vi "CreateSwapArray_v2.vi"(8 "error in (no error)":errorcluster, 9 "ROSCO Params":T3, 10 "Index In":T2={"iSTATUS"=0, "TIME"=0, "DT"=0, "BL_PITCH_1"=0, "VS_MECHGENPWR"=13, "GEN_SPEED"=0, "ROT_SPEED"=0, "GENTQMEAS"=0, "Y_M"=0, "HORWINDV"=0, "ROOTMOOP1"=0, "ROOTMOOP2"=0, "BL_PITCH_2"=0, "BL_PITCH_3"=0, "ROOTMOOP3"=0, "INFILE_SIZE"=0, "FA_ACC"=0, "NUM_BLADES"=0, " OUT BL_PITCH"=0, "OUT_ TORQUE"=0, "OUTFILE_SIZE "=0, "AVCMSG_SIZE"=0, "AERODYN TQ"=46, "VS_GENPWR"=0}, 11 "SwapIn":T1) -> (0 "error out":errorcluster, 1 "ROSCO Params Out":T3, 2 "Index Out":T2={"iSTATUS"=0, "TIME"=0, "DT"=0, "BL_PITCH_1"=0, "VS_MECHGENPWR"=13, "GEN_SPEED"=0, "ROT_SPEED"=0, "GENTQMEAS"=0, "Y_M"=0, "HORWINDV"=0, "ROOTMOOP1"=0, "ROOTMOOP2"=0, "BL_PITCH_2"=0, "BL_PITCH_3"=0, "ROOTMOOP3"=0, "INFILE_SIZE"=0, "FA_ACC"=0, "NUM_BLADES"=0, " OUT BL_PITCH"=0, "OUT_ TORQUE"=0, "OUTFILE_SIZE "=0, "AVCMSG_SIZE"=0, "AERODYN TQ"=46, "VS_GENPWR"=0}, 3 "SwapIn Out":T1, 4 "avrSWAP":sgl[](array[numeric]))   [LabVIEW 2018]
uses:
  Clusters/SwapIn.ctl
  Clusters/SwapIndexes.ctl
  Clusters/RoscoParams.ctl
  Clusters/ArrayPairs.ctl
  Clusters/SwapArrayCluster.ctl
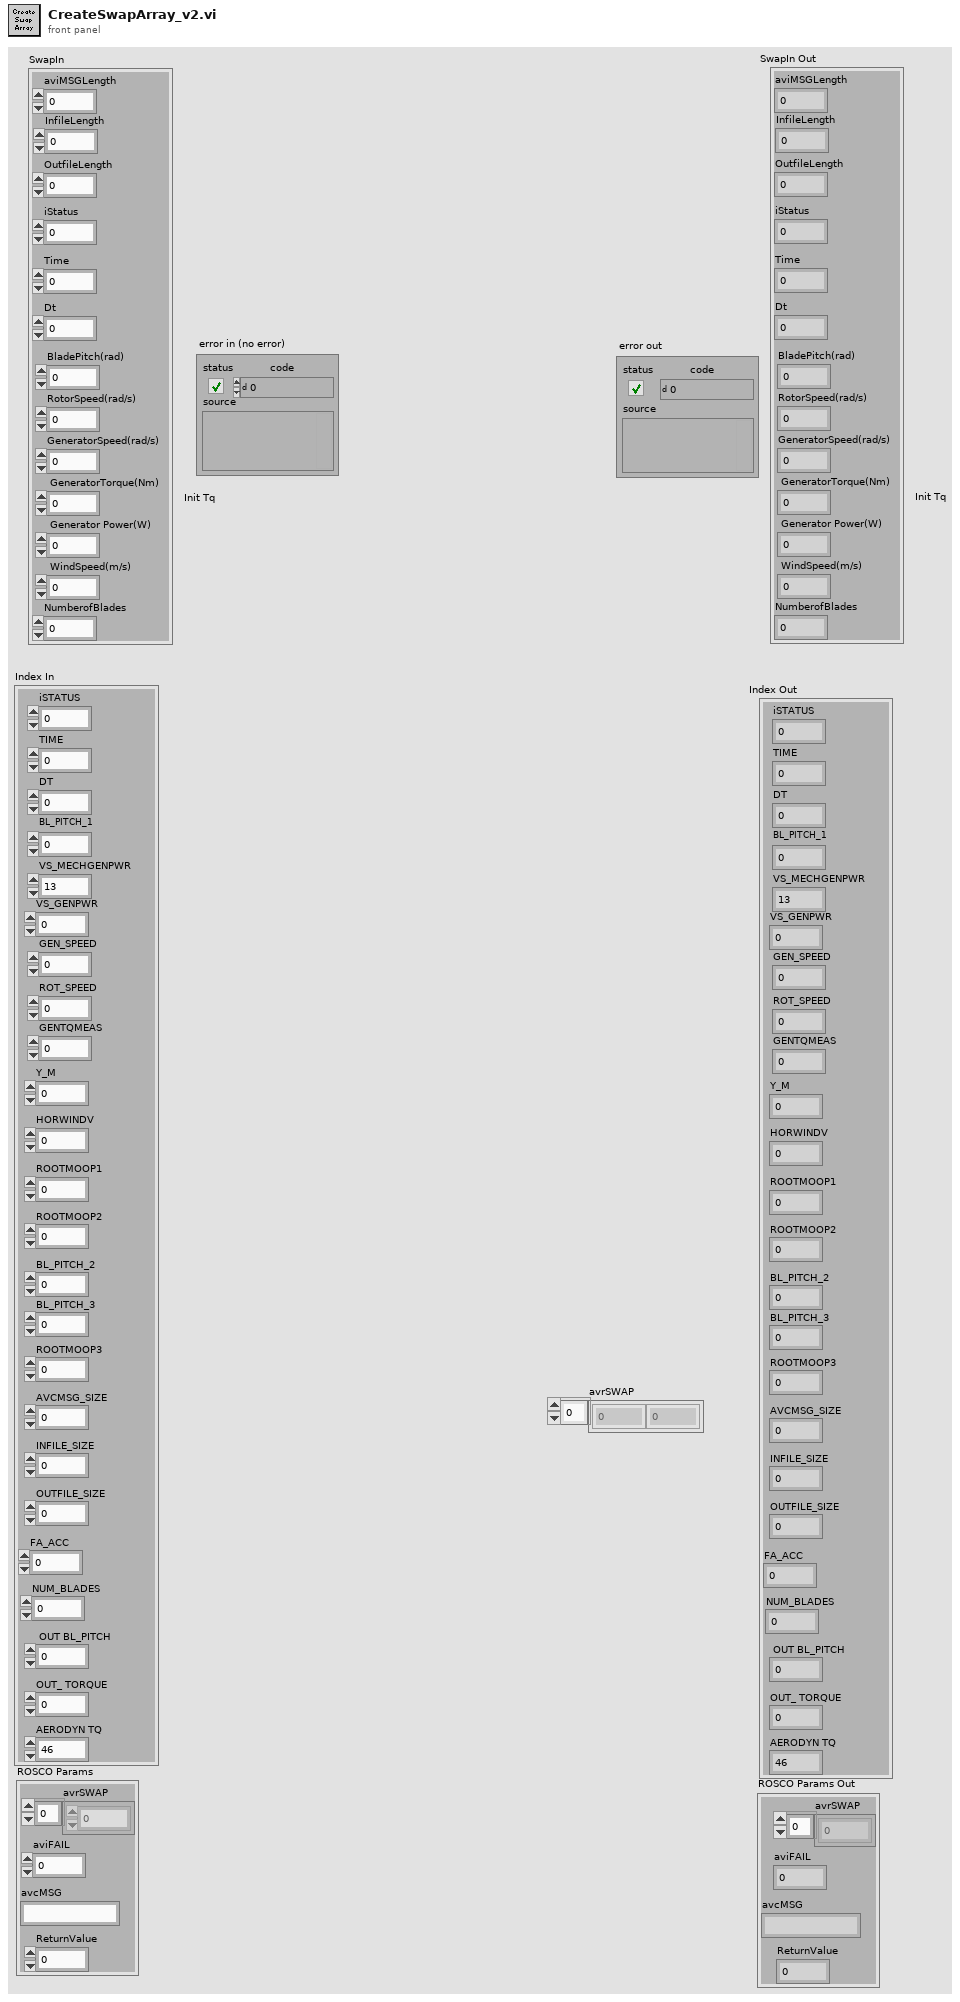
[diagram p1: front panel]
types:
  T1 = typedef "SwapIn.ctl" = cluster{"BladePitch(rad)":sgl, "RotorSpeed(rad/s)":sgl, "GeneratorSpeed(rad/s)":sgl, " GeneratorTorque(Nm)":sgl, " Generator Power(W) ":sgl, " WindSpeed(m/s)":sgl, "aviMSGLength":sgl, "InfileLength":sgl, "OutfileLength":sgl, "iStatus":sgl, "Time":sgl, "Dt":sgl, "NumberofBlades":sgl}
  T2 = typedef "SwapIndexes.ctl" = cluster{"iSTATUS":i32, "TIME":i32, "DT":i32, "BL_PITCH_1":i32, "VS_MECHGENPWR":i32, "GEN_SPEED":i32, "ROT_SPEED":i32, "GENTQMEAS":i32, "Y_M":i32, "HORWINDV":i32, "ROOTMOOP1":i32, "ROOTMOOP2":i32, "BL_PITCH_2":i32, "BL_PITCH_3":i32, "ROOTMOOP3":i32, "INFILE_SIZE":i32, "FA_ACC":i32, "NUM_BLADES":i32, " OUT BL_PITCH":i32, "OUT_ TORQUE":i32, "OUTFILE_SIZE ":i32, "AVCMSG_SIZE":i32, "AERODYN TQ":i32, "VS_GENPWR":i32}
  T3 = typedef "RoscoParams.ctl" = cluster{"avrSWAP":sgl[], "aviFAIL":i32, "avcMSG":string, "ReturnValue":i32}
  T4 = typedef "ArrayPairs.ctl" = cluster{"iStatus":T5, "TIME":T5, "DT":T5, "BL_PITCH":T5, "VS_MECHGENPWR":T5, "VS_GENPWR":T5, "GEN_SPEED":T5, "ROTOR_SPEED":T5, "GENTQMEAS":T5, "Y_M":T5, "HORWINDV":T5, "ROOTMOOP1":T5, "ROOTMOOP2":T5, "BL_PITCH2":T5, "BL_PITCH3":T5, "ROOTMOOP3":T5, "AVCMSG_SIZE":T5, "INFILE_SIZE ":T5, "OUTFILE_SIZE ":T5, "FA_ACC":T5, "NUM_BLADES":T5, "OUT_BL_PITCH":T5, "OUT_TORQUE":T5, "OUT_AERODYN_TQ":T5}
  T5 = typedef "SwapArrayCluster.ctl" = cluster{"Index":i32, "Value":sgl}
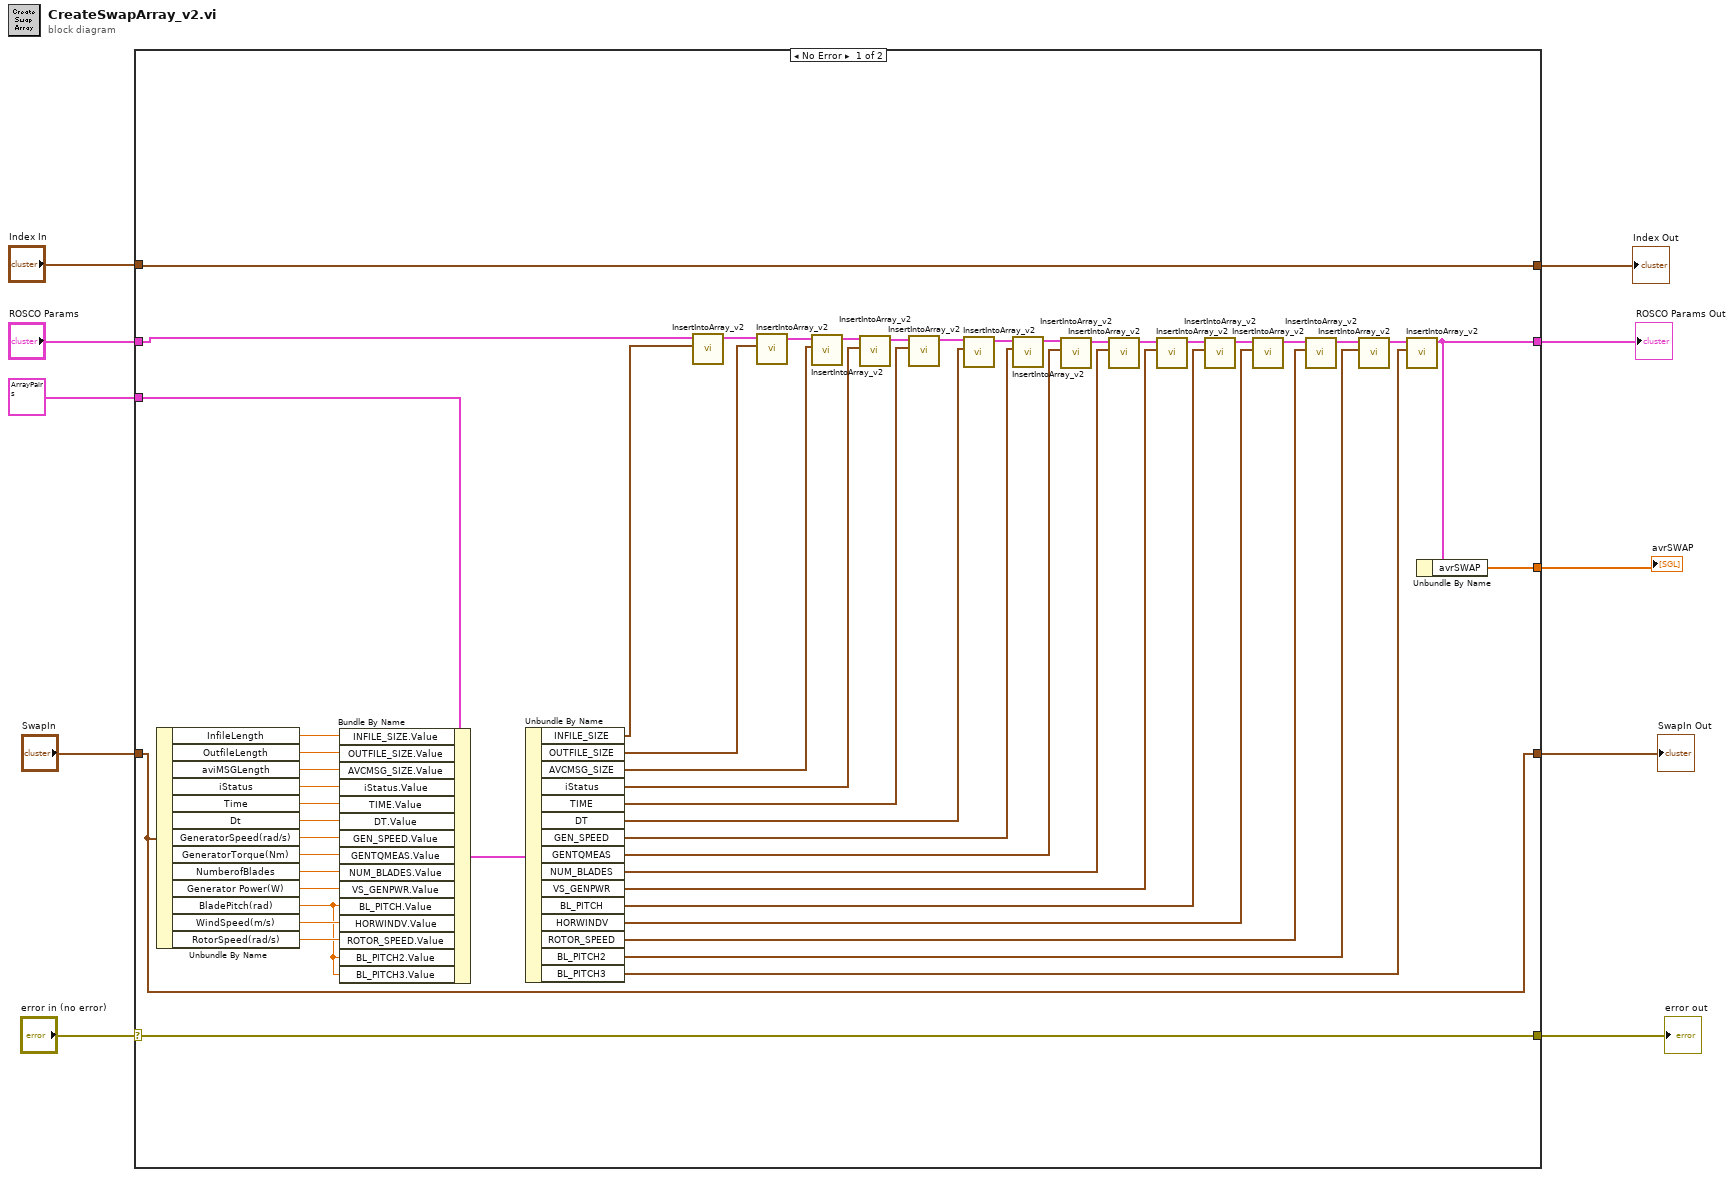
[diagram p0: block diagram]
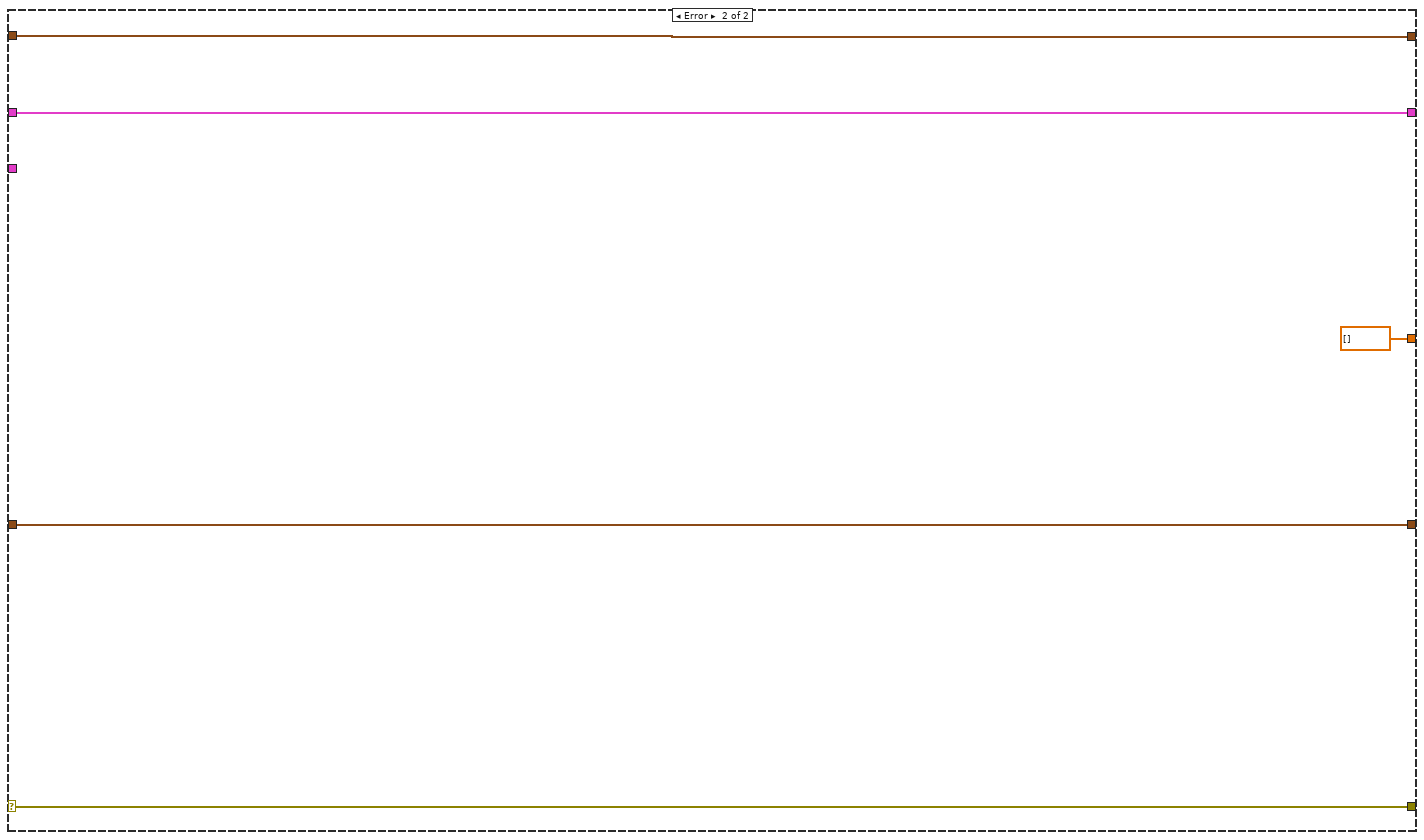
[diagram p2: hidden frame]
diagram:
  n1 = case shown="No Error" "error in (no error)" {
    selector: "error in (no error)" -> [w17 w62]
    tunnel: "SwapIn" -> [w59 w63]
    tunnel: "Index In" -> [w60 w64]
    tunnel: "ROSCO Params" -> [w46 w65]
    tunnel: [w60 w64] -> w7
    tunnel: [w11 w65] -> w6
    tunnel: [w59 w63] -> w5
    tunnel: T4 {"iStatus"={"Index"=0, "Value"=0.0}, "TIME"={"Index"=1, "Value"=0.0}, "DT"={"Index"=2, "Value"=0.0}, "BL_PITCH"={"Index"=3, "Value"=0.0}, "VS_MECHGENPWR"={"Index"=13, "Value"=0.0}, "VS_GENPWR"={"Index"=14, "Value"=0.0}, "GEN_SPEED"={"Index"=19, "Value"=0.0}, "ROTOR_SPEED"={"Index"=20, "Value"=0.0}, "GENTQMEAS"={"Index"=22, "Value"=0.0}, "Y_M"={"Index"=23, "Value"=0.0}, "HORWINDV"={"Index"=26, "Value"=0.0}, "ROOTMOOP1"={"Index"=29, "Value"=0.0}, "ROOTMOOP2"={"Index"=30, "Value"=0.0}, "BL_PITCH2"={"Index"=32, "Value"=0.0}, "BL_PITCH3"={"Index"=33, "Value"=0.0}, "ROOTMOOP3"={"Index"=31, "Value"=0.0}, "AVCMSG_SIZE"={"Index"=48, "Value"=0.0}, "INFILE_SIZE "={"Index"=49, "Value"=0.0}, "OUTFILE_SIZE "={"Index"=50, "Value"=0.0}, "FA_ACC"={"Index"=52, "Value"=0.0}, "NUM_BLADES"={"Index"=60, "Value"=0.0}, "OUT_BL_PITCH"={"Index"=44, "Value"=0.0}, "OUT_TORQUE"={"Index"=46, "Value"=0.0}, "OUT_AERODYN_TQ"={"Index"=89, "Value"=0.0}} ("ArrayPairs") -> [w45 _]
    tunnel: [w17 w62] -> w3
    tunnel: [w18 sgl[] [] ("avrSWAP")] -> w1
    frame No Error {
      n2 = Unbundle By Name(w59) -> ("InfileLength"=w47:sgl, "OutfileLength"=w48:sgl, "aviMSGLength"=w49:sgl, "iStatus"=w50:sgl, "Time"=w51:sgl, "Dt"=w52:sgl, "GeneratorSpeed(rad/s)"=w53:sgl, "GeneratorTorque(Nm)"=w54:sgl, "NumberofBlades"=w55:sgl, "Generator Power(W)"=w56:sgl, "BladePitch(rad)"=w16:sgl, "WindSpeed(m/s)"=w57:sgl, "RotorSpeed(rad/s)"=w58:sgl)
      n3 = Bundle By Name(cluster=w45, "INFILE_SIZE.Value"=w47, "OUTFILE_SIZE.Value"=w48, "AVCMSG_SIZE.Value"=w49, "iStatus.Value"=w50, "TIME.Value"=w51, "DT.Value"=w52, "GEN_SPEED.Value"=w53, "GENTQMEAS.Value"=w54, "NUM_BLADES.Value"=w55, "VS_GENPWR.Value"=w56, "BL_PITCH.Value"=w16, "HORWINDV.Value"=w57, "ROTOR_SPEED.Value"=w58, "BL_PITCH2.Value"=w16, "BL_PITCH3.Value"=w16) -> (w44:T4)
      n4 = Unbundle By Name(w44) -> ("INFILE_SIZE"=w43:T5, "OUTFILE_SIZE"=w37:T5, "AVCMSG_SIZE"=w35:T5, "iStatus"=w34:T5, "TIME"=w33:T5, "DT"=w26:T5, "GEN_SPEED"=w25:T5, "GENTQMEAS"=w24:T5, "NUM_BLADES"=w23:T5, "VS_GENPWR"=w22:T5, "BL_PITCH"=w21:T5, "HORWINDV"=w20:T5, "ROTOR_SPEED"=w19:T5, "BL_PITCH2"=w15:T5, "BL_PITCH3"=w14:T5)
      n5 = call "InsertIntoArray_v2.vi"("ROSCO Params"=w46, "KeyVal"=w43) -> ("ROSCO Params Out"=w42:T3)  [unwired: 7 in, 1 out]
      n6 = call "InsertIntoArray_v2.vi"("ROSCO Params"=w42, "KeyVal"=w37) -> ("ROSCO Params Out"=w36:T3)  [unwired: 7 in, 1 out]
      n7 = call "InsertIntoArray_v2.vi"("ROSCO Params"=w36, "KeyVal"=w35) -> ("ROSCO Params Out"=w32:T3)  [unwired: 7 in, 1 out]
      n8 = call "InsertIntoArray_v2.vi"("ROSCO Params"=w32, "KeyVal"=w34) -> ("ROSCO Params Out"=w41:T3)  [unwired: 7 in, 1 out]
      n9 = call "InsertIntoArray_v2.vi"("ROSCO Params"=w41, "KeyVal"=w33) -> ("ROSCO Params Out"=w31:T3)  [unwired: 7 in, 1 out]
      n10 = call "InsertIntoArray_v2.vi"("ROSCO Params"=w31, "KeyVal"=w26) -> ("ROSCO Params Out"=w40:T3)  [unwired: 7 in, 1 out]
      n11 = call "InsertIntoArray_v2.vi"("ROSCO Params"=w40, "KeyVal"=w25) -> ("ROSCO Params Out"=w30:T3)  [unwired: 7 in, 1 out]
      n12 = call "InsertIntoArray_v2.vi"("ROSCO Params"=w30, "KeyVal"=w24) -> ("ROSCO Params Out"=w39:T3)  [unwired: 7 in, 1 out]
      n13 = call "InsertIntoArray_v2.vi"("ROSCO Params"=w39, "KeyVal"=w23) -> ("ROSCO Params Out"=w29:T3)  [unwired: 7 in, 1 out]
      n14 = call "InsertIntoArray_v2.vi"("ROSCO Params"=w29, "KeyVal"=w22) -> ("ROSCO Params Out"=w28:T3)  [unwired: 7 in, 1 out]
      n15 = call "InsertIntoArray_v2.vi"("ROSCO Params"=w28, "KeyVal"=w21) -> ("ROSCO Params Out"=w38:T3)  [unwired: 7 in, 1 out]
      n16 = call "InsertIntoArray_v2.vi"("ROSCO Params"=w38, "KeyVal"=w20) -> ("ROSCO Params Out"=w27:T3)  [unwired: 7 in, 1 out]
      n17 = call "InsertIntoArray_v2.vi"("ROSCO Params"=w27, "KeyVal"=w19) -> ("ROSCO Params Out"=w13:T3)  [unwired: 7 in, 1 out]
      n18 = call "InsertIntoArray_v2.vi"("ROSCO Params"=w13, "KeyVal"=w15) -> ("ROSCO Params Out"=w12:T3)  [unwired: 7 in, 1 out]
      n19 = call "InsertIntoArray_v2.vi"("ROSCO Params"=w12, "KeyVal"=w14) -> ("ROSCO Params Out"=w11:T3)  [unwired: 7 in, 1 out]
      n20 = Unbundle By Name(w11) -> ("avrSWAP"=w18:sgl[])
    }
    frame Error {
    }
  }
  "error out" <- w3
  "SwapIn Out" <- w5
  "Index Out" <- w7
  "ROSCO Params Out" <- w6
  "avrSWAP" <- w1
